vi "Process.vi"(8 "error in":errorcluster, 11 "SMO.TimedLoop":refnum<class "SMO.TimedLoop.lvclass">) -> (0 "error out":errorcluster, 3 "SMO.TimedLoop out":refnum<class "SMO.TimedLoop.lvclass">)   [LabVIEW 2013, in "SMO.TimedLoop.lvclass"]
doc: "---------------------------------------------------------------\nJKI State Machine Objects™\nhttp://jki.net/state-machine-objects/\nCopyright (C) 2005-2015, JKI <info@jki.net>\nALL RIGHTS RESERVEDJKI State Machine Objects (SMO) 1.0.0.5\nJKI - JKI\nCopyright (c) 2016, JKI"
uses:
  SMO.TimedLoop.lvclass
  <vilib>/JKI/JKI SMO/SMO/Typedefs/Parent Call--Enum.ctl
  <vilib>/JKI/JKI SMO/SMO/SMO.lvclass
  <vilib>/Platform/TimedLoop/XDataNode/timing_clust.ctl
  <vilib>/Platform/TimedLoop/XDataNode/nitl_modes.ctl
  <vilib>/Platform/TimedLoop/XDataNode/wakeup.ctl
  <vilib>/platform/TimedLoop/XDataNode/XDataNode.xnode
  <vilib>/Platform/TimedLoop/XDataNode/XDNodeRunTimeDep.lvlib
panel:
  # "For instructions on how to use the JKI State Machine Objects, examples and video tutorials, visit:\nhttp://jki.net/state-machine-objects/\n\nJKI State Machine Objects™\nhttp://jki.net/state-machine-objects/\nCopyright (C) 2005-2015, JKI <info@jki.net>\nALL RIGHTS RESERVED"
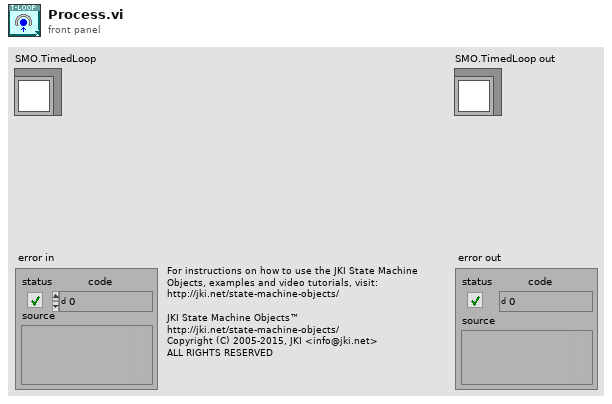
[diagram p1: front panel]
types:
  T1 = typedef "SMO.lvclass/Parent Call--Enum.ctl" = enum16{"Allows parent to run", "Does not request parent to run"}
  T2 = typedef "XDNodeRunTimeDep.lvlib/timing_clust.ctl" = cluster{"Expected End [f-1]":u64, "Actual End [f-1]":u64, "Finished Late? [f-1]":bool, "Expected End [i-1]":u64, "Actual End [i-1]":u64, "Finished Late? [i-1]":bool, "Expected Start [i]":u64, "Actual Start [i]":u64, "Expected Start [f]":u64, "Actual Start [f]":u64, "Source Name":string, "Structure Name":string, "Period":i64, "Deadline":i64, "Offset":i64, "Start":i64, "Priority":i32, "Timeout":i32, "Mode":T3, "Wakeup Reason":T4, "Error":errorcluster, "Source Type":string, "Secondary Source Type":string, "Global End Time":u64, "Global Start Time":u64, "Frame Duration":u64, "Iteration Duration":u64, "Assigned CPU":i32, "I/O Scan Engine Mode":u32}
  T3 = typedef "XDNodeRunTimeDep.lvlib/nitl_modes.ctl" = enum32{"No Change", "Process missed periods, maintain original phase", "Discard missed periods, maintain original phase", "Process missed periods, ignore original phase", "Discard missed periods, ignore original phase"}
  T4 = typedef "XDNodeRunTimeDep.lvlib/wakeup.ctl" = enum32{"Normal", "Aborted", "Asynchronous wakeup", "Timing source error", "Timed loop error", "Timeout"}
  T5 = typedef "SMO.TimedLoop.lvclass/PrivateEvents--Cluster.ctl" = cluster{"AsyncMethod":refnum<user-event>}
  T6 = typedef "SMO.lvclass/Protected Events.ctl" = cluster{"StopProcesses":refnum<user-event>, "AbortProcesses":refnum<user-event>, "Config Changed":refnum<user-event>}
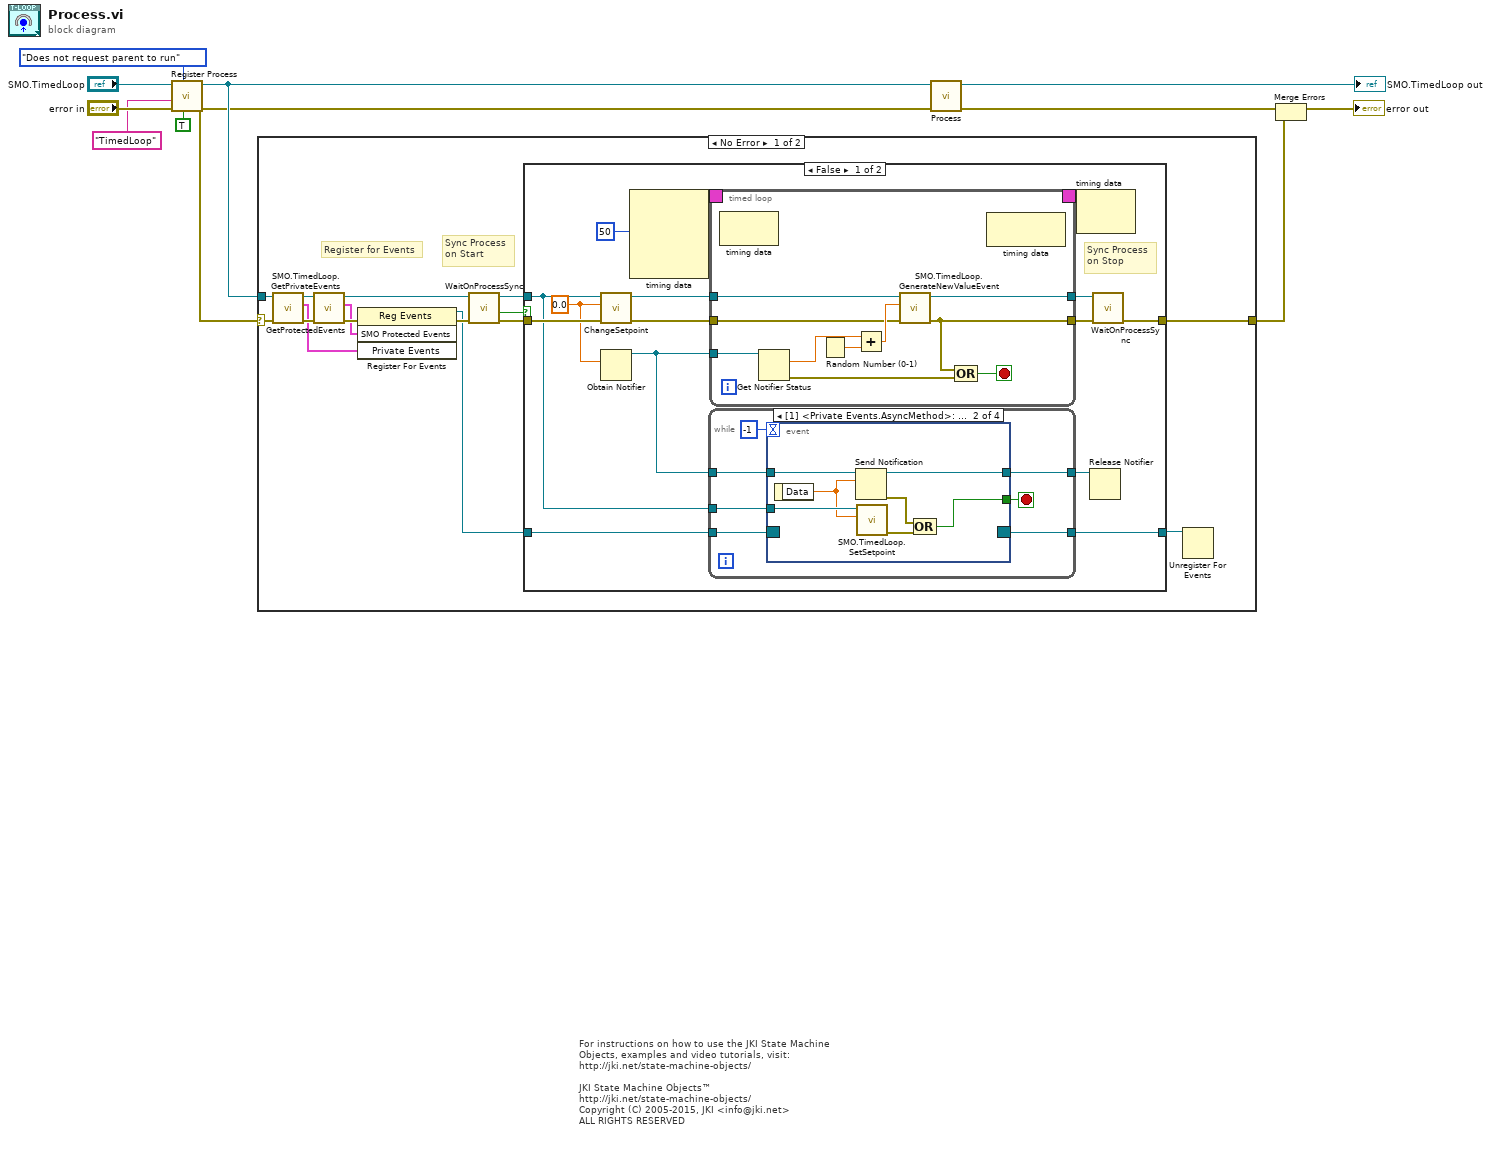
[diagram p0: block diagram]
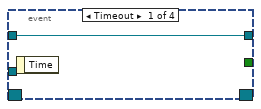
[diagram p2: hidden frame]
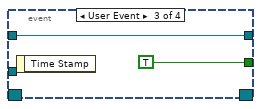
[diagram p3: hidden frame]
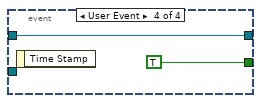
[diagram p4: hidden frame]
diagram:
  # "For instructions on how to use the JKI State Machine Objects, examples and video tutorials, visit:\nhttp://jki.net/state-machine-objects/\n\nJKI State Machine Objects™\nhttp://jki.net/state-machine-objects/\nCopyright (C) 2005-2015, JKI <info@jki.net>\nALL RIGHTS RESERVED"
  n1 = call <vilib>:"Register Process.vi"("Forces Self to Run (F)"=TRUE, "Parent Call"=Parent_Call--Enum."Does not request parent to run", "error in (no error)"="error in", "Process Name (optional)"="TimedLoop", "SMO"="SMO.TimedLoop") -> ("error out"=w1:errorcluster, "SMO out"=w2:refnum<class "SMO.TimedLoop.lvclass">)  [unwired: 5 in]
  n2 = case shown="No Error" w1 {
    selector: w1 -> [w14 w79]
    tunnel: w2 -> [w16 _]
    tunnel: [w18 w79] -> w6
    frame No Error {
      # "Sync Process\non Start"
      # "Register for Events"
      n3 = call "SMO.TimedLoop.GetPrivateEvents.vi"("error in (no error)"=w14, "SMO.TimedLoop"=w16) -> ("error out"=w13:errorcluster, "Private Events"=w12:T5, "SMO.TimedLoop out"=w15:refnum<class "SMO.TimedLoop.lvclass">)  [unwired: 7 in]
      n4 = call <vilib>:"GetProtectedEvents.vi"("error in (no error)"=w13, "SMO"=w15) -> ("error out"=w21:errorcluster, "SMO Protected Events"=w20:T6, "SMO out"=w22:refnum<class "SMO.TimedLoop.lvclass">)  [unwired: 7 in]
      n5 = register-events(error in=w21, w20, w12) -> (reference out=w19:refnum<event-registration>, error out=w23:errorcluster)  [unwired: 1 in]
      n6 = call <vilib>:"WaitOnProcessSync.vi"("error in (no error)"=w23, "SMO"=w22) -> ("error out"=w25:errorcluster, "Don't run?"=w26:bool, "SMO out"=w24:refnum<class "SMO.TimedLoop.lvclass">)  [unwired: 7 in]
      n7 = case shown="False" w26 {
        tunnel: w25 -> [w32 w77]
        tunnel: w24 -> [w27 _]
        tunnel: w19 -> [w35 w78]
        tunnel: [w36 w77] -> w18
        tunnel: [w34 w78] -> w17
        frame False {
          w29 = 0.0 ("Setpoint")
          # "Sync Process\non Stop"
          n8 = call "ChangeSetpoint.vi"("error in (no error)"=w32, "Setpoint"=w29, "SMO.TimedLoop"=w27) -> ("error out"=w31:errorcluster, "SMO.TimedLoop out"=w30:refnum<class "SMO.TimedLoop.lvclass">)  [unwired: 7 in]
          n9 = Obtain Notifier(notification data type=w29) -> (notifier out=w28:refnum<notifier>)  [unwired: 3 in, 2 out]
          n10 = node-c288(i64 50 ("Period")) -> (w41:T2)  [unwired: 3 in]
          n11 = while {
            tunnel: w35 -> [w47]
            tunnel: [w46] -> w34
            tunnel: [w43] -> w33
            tunnel: w28 -> [w44]
            tunnel: w27 -> [w42]
            stop <- w45 stop-if-true
            n12 = event shown="[1] <Private Events.AsyncMethod>: User Event" {
              selector: w47 -> [_ _ _ _]
              dyn-events: [_ _ _ _] -> w46
              timeout: -1 -> [_ _ _ _]
              tunnel: [_ w50 TRUE TRUE] -> w45
              tunnel: w44 -> [w49 w56 w57 w59]
              tunnel: [w49 w55 w57 w59] -> w43
              tunnel: w42 -> [_ w54 _ _]
              event Timeout {
                n13 = event-data() -> ()  [unwired: 1 in, 1 out]
              }
              event User Event {
                n14 = event-data() -> ("Data"=w53:dbl)  [unwired: 1 in]
                n15 = Send Notification(notification=w53, notifier=w56) -> (notifier out=w55:refnum<notifier>, error out=w51:errorcluster)  [unwired: 1 in]
                n16 = call "SMO.TimedLoop.SetSetpoint.vi"("Setpoint"=w53, "SMO.TimedLoop"=w54) -> ("error out"=w52:errorcluster)  [unwired: 8 in, 1 out]
                n17 = Compound Arithmetic op=OR(w51, w52) -> (w50:bool)
              }
              event User Event {
                n18 = event-data() -> ()  [unwired: 1 in, 1 out]
              }
              event User Event {
                n19 = event-data() -> ()  [unwired: 1 in, 1 out]
              }
            }
          }
          n20 = timed-loop {
            timing: w41 -> [_]
            timing-out: [_] -> w40
            tunnel: w30 -> [w62]
            tunnel: w31 -> [w61]
            tunnel: w28 -> [w70]
            tunnel: [w67] -> w38
            tunnel: [w66] -> w37
            stop <- w68 stop-if-true
            n21 = node-c288() -> ()  [unwired: 1 in, 1 out]
            n22 = Get Notifier Status(notifier=w70) -> (current notification=w63:dbl, error out=w69:errorcluster)  [unwired: 1 in, 3 out]
            n23 = Random Number (0-1)() -> (number: 0 to 1=w65:dbl)
            n24 = Add(x=w63, y=w65) -> (x+y=w64:dbl)
            n25 = call "SMO.TimedLoop.GenerateNewValueEvent.vi"("error in (no error)"=w61, "New Value"=w64, "SMO.TimedLoop"=w62) -> ("error out"=w66:errorcluster, "SMO.TimedLoop out"=w67:refnum<class "SMO.TimedLoop.lvclass">)  [unwired: 7 in]
            n26 = Compound Arithmetic op=OR(w66, w69) -> (w68:bool)
            n27 = node-c288() -> ()  [unwired: 1 in, 1 out]
          }
          n28 = node-c288(w40) -> ()  [unwired: 1 out]
          n29 = Release Notifier(notifier=w33) -> ()  [unwired: 2 in, 3 out]
          n30 = call <vilib>:"WaitOnProcessSync.vi"("error in (no error)"=w37, "SMO"=w38) -> ("error out"=w36:errorcluster)  [unwired: 7 in, 2 out]
        }
        frame True {
        }
      }
      n31 = Unregister For Events(event registration refnum=w17) -> ()  [unwired: 1 in, 1 out]
    }
    frame Error {
    }
  }
  n32 = call-parent "Process.vi"("error in"=w1, "SMO"=w2) -> ("error out"=w7:errorcluster, "SMO out"=→"SMO.TimedLoop out":refnum<class "SMO.TimedLoop.lvclass">)  [unwired: 8 in]
  n33 = Merge Errors(w7, w6) -> (→"error out":errorcluster)
